vi "SetupMovieSlide.vi"(1 "Name":string, 2 "Template":path=path "/Kim/Users/crogers/Dropbox/LVPresent/Templates/MovieTemplate.vi") -> (0 "success?":bool)   [LabVIEW 2012]
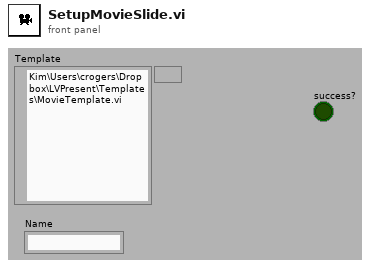
[diagram p1: front panel]
types:
  T1 = typedef "QT_Ref.ctl" = refnum<k1>
  T2 = typedef "QT_Image.ctl" = cluster{"Width":i32, "Height":i32, "Depth":i32, "data":u8[], "Compressed data":u8[], "Color table":u32[], "Duration":i32, "Options":i32, "Timestamp":i32, "ID":i32, "Reserved":i32, "Dialogs":u32}
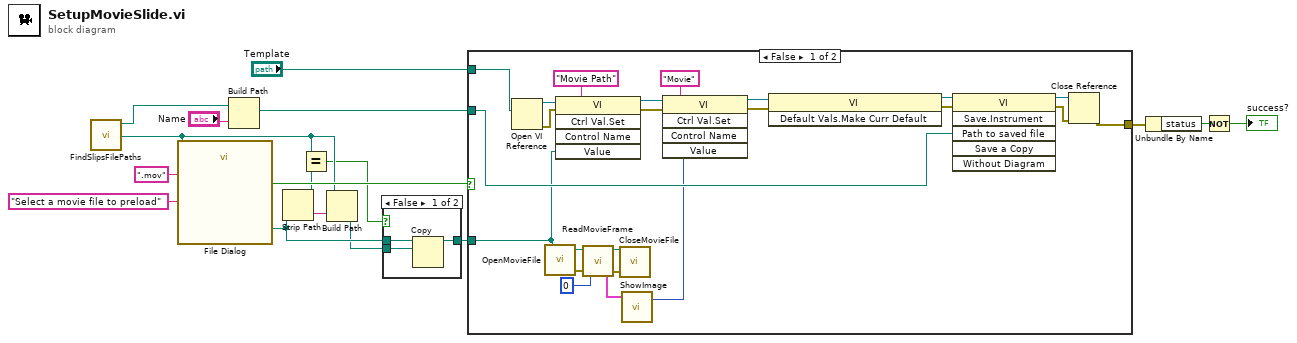
[diagram p0: block diagram]
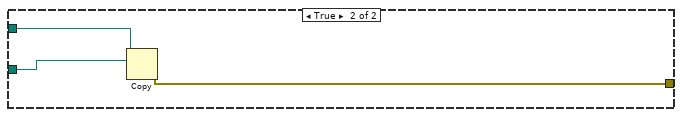
[diagram p3: hidden frame]
diagram:
  n1 = call "FindSlipsFilePaths.vi"() -> ("Movies"=w9:path, "Slides"=w14:path)  [unwired: 2 in, 3 out]
  n2 = call "File Dialog"("start path"=w9, "prompt"="Select a movie file to preload", "pattern (all files)"=".mov") -> ("selected path"=w7:path, "cancelled"=w15:bool)  [unwired: 9 in, 2 out]
  n3 = Build Path(base path=w14, name or relative path="Name") -> (appended path=w12:path)
  n4 = Strip Path(path=w7) -> (stripped path=w11:path, name=w10:string)
  n5 = Equal?(x=w9, y=w11) -> (x = y?=w8:bool)
  n6 = Build Path(base path=w9, name or relative path=w10) -> (appended path=w6:path)
  n7 = case shown="False" w8 {
    tunnel: w7 -> [w20 w21]
    tunnel: w6 -> [w19 _]
    tunnel: [w18 w21] -> w5
    frame False {
      n8 = Copy(10:w19, 11:w20) -> (3:w18:path)  [unwired: 3 in, 2 out]
    }
    frame True {
    }
  }
  n9 = case shown="False" w15 {
    tunnel: w12 -> [w37 w46]
    tunnel: w5 -> [w25 _]
    tunnel: "Template" -> [w23 w47]
    tunnel: [w22 w45] -> w3
    frame False {
      n10 = Open VI Reference(vi path=w23) -> (vi reference=w44:refnum<vi>, error out=w43:errorcluster)  [unwired: 5 in]
      n11 = call <userlib>:"OpenMovieFile.vi"("Path"=w25) -> ("error out"=w26:errorcluster, "QT Ref Out"=w27:T1)  [unwired: 1 out]
      n12 = invoke class="VI" method="Ctrl Val.Set"(reference=w44, error in=w43, "Control Name"="Movie Path", "Value"=w25) -> (reference out=w36:refnum<vi>, error out=w35:errorcluster)  [unwired: 1 in, 3 out]
      n13 = call <userlib>:"ReadMovieFrame.vi"("error in"=w26, "Frame Number"=0, "QT Ref In"=w27) -> ("error out"=w28:errorcluster, "Image Out"=w30:T2, "QT Ref Out"=w29:T1)
      n14 = call <userlib>:"CloseMovieFile.vi"("error out"=w28, "QT Ref Out"=w29) -> ()  [unwired: 2 in]
      n15 = call <userlib>:"ShowImage.vi"("Image"=w30) -> ("image"=w24:picture)  [unwired: 2 in, 1 out]
      n16 = invoke class="VI" method="Ctrl Val.Set"(reference=w36, error in=w35, "Control Name"="Movie", "Value"=w24) -> (reference out=w33:refnum<vi>, error out=w34:errorcluster)  [unwired: 1 in, 3 out]
      n17 = invoke class="VI" method="Default Vals.Make Curr Default"(reference=w33, error in=w34) -> (reference out=w41:refnum<vi>, error out=w40:errorcluster)  [unwired: 1 in, 1 out]
      n18 = invoke class="VI" method="Save.Instrument"(reference=w41, error in=w40, "Path to saved file"=w37) -> (reference out=w38:refnum<vi>, error out=w39:errorcluster)  [unwired: 3 in, 4 out]
      n19 = Close Reference(reference=w38, error in (no error)=w39) -> (error out=w22:errorcluster)
    }
    frame True {
      n20 = Copy(10:w46, 11:w47) -> (0:w45:errorcluster)  [unwired: 3 in, 2 out]
    }
  }
  n21 = Unbundle By Name(w3) -> ("status"=w2:bool)
  n22 = Not(x=w2) -> (.not. x?=→"success?":bool)
